vi "Manual Test.vi"() -> ()   [LabVIEW 2019]
uses:
  <vilib>/Gustavo Trejo/PIC Serial Toolkit/Controls/TRISA.ctl
  <vilib>/Gustavo Trejo/PIC Serial Toolkit/Controls/TRISB.ctl
  <vilib>/Gustavo Trejo/PIC Serial Toolkit/Controls/TRISC.ctl
  <vilib>/Gustavo Trejo/PIC Serial Toolkit/Controls/TRISD.ctl
  <vilib>/Gustavo Trejo/PIC Serial Toolkit/Controls/TRISE.ctl
  <vilib>/Gustavo Trejo/PIC Serial Toolkit/Controls/Pin Number.ctl
panel:
  in  "D5":bool
  in  "D4":bool
  out "D3":bool
  out "D2":bool
  in  "Stop Button":bool
  in  "COM":refnum<visa-resource-name>
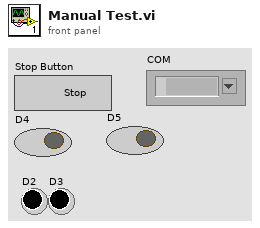
[diagram p1: front panel]
types:
  T1 = typedef "TRISE.ctl" = cluster{"E0":bool, "E1":bool, "E2":bool}
  T2 = typedef "TRISD.ctl" = cluster{"D0":bool, "D1":bool, "D2":bool, "D3":bool, "D4":bool, "D5":bool, "D6":bool, "D7":bool}
  T3 = typedef "TRISC.ctl" = cluster{"C0":bool, "C1":bool, "C2":bool, "C3":bool, "C4":bool, "C5":bool}
  T4 = typedef "TRISB.ctl" = cluster{"B0":bool, "B1":bool, "B2":bool, "B3":bool, "B4":bool, "B5":bool, "B6":bool, "B7":bool}
  T5 = typedef "TRISA.ctl" = cluster{"A0":bool, "A1":bool, "A2":bool, "A3":bool, "A4":bool, "A5":bool, "A6":bool, "A7":bool}
  T6 = typedef "Pin Number.ctl" = enum16{"A0/AN0", "A1/AN1", "A2/AN2", "A3/AN3", "A4", "A5/AN4", "A6", "A7", "B0/AN12", "B1/AN10", "B2/AN8", "B3/AN9", "B4/AN11", "B5/AN13", "B6", "B7", "C0", "C1/PWM2", "C2/PWM1", "C3", "C4", "C5", "D0", "D1", "D2", "D3", "D4", "D5", "D6", "D7", "E0/AN5", "E1/AN6", "E2/AN7"}
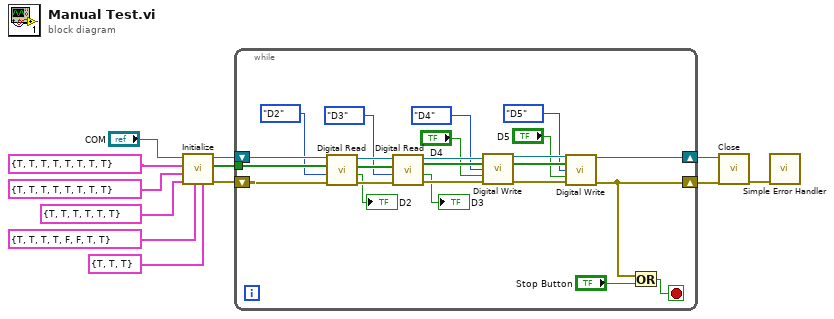
[diagram p0: block diagram]
diagram:
  n1 = call <vilib>:"Initialize.vi"("TRISE E0-E2"=T1 {"E0"=TRUE, "E1"=TRUE, "E2"=TRUE}, "TRISD D0-D7"=T2 {"D0"=TRUE, "D1"=TRUE, "D2"=TRUE, "D3"=TRUE, "D4"=FALSE, "D5"=FALSE, "D6"=TRUE, "D7"=TRUE}, "TRISC C0-C5"=T3 {"C0"=TRUE, "C1"=TRUE, "C2"=TRUE, "C3"=TRUE, "C4"=TRUE, "C5"=TRUE}, "TRISB B0-B7"=T4 {"B0"=TRUE, "B1"=TRUE, "B2"=TRUE, "B3"=TRUE, "B4"=TRUE, "B5"=TRUE, "B6"=TRUE, "B7"=TRUE}, "TRISA A0-A7"=T5 {"A0"=TRUE, "A1"=TRUE, "A2"=TRUE, "A3"=TRUE, "A4"=TRUE, "A5"=TRUE, "A6"=TRUE, "A7"=TRUE}, "VISA Refnum in"="COM") -> ("error out"=w4:errorcluster, "Ports Ref Out"=w5:bool[], "VISA Refnum out"=w6:refnum<visa-resource-name>)  [unwired: 3 in]
  n2 = while {
    tunnel: w5 -> [w35]
    shift-right: [w13] -> w2
    shift-left: w6 -> [w36]
    shift-right: [w14] -> w3
    shift-left: w4 -> [w34]
    stop <- w23 stop-if-true
    n3 = call <vilib>:"Digital Read.vi"("error in (no error)"=w34, "Pin Number"=Pin_Number."D2", "Ports Ref In"=w35, "VISA Refnum in"=w36) -> ("error out"=w33:errorcluster, "Pin State Out"=→"D2":bool, "Ports Ref Out"=w32:bool[], "VISA Refnum out"=w31:refnum<visa-resource-name>)  [unwired: 4 in]
    n4 = call <vilib>:"Digital Read.vi"("error in (no error)"=w33, "Pin Number"=Pin_Number."D3", "Ports Ref In"=w32, "VISA Refnum in"=w31) -> ("error out"=w30:errorcluster, "Pin State Out"=→"D3":bool, "Ports Ref Out"=w28:bool[], "VISA Refnum out"=w29:refnum<visa-resource-name>)  [unwired: 4 in]
    n5 = call <vilib>:"Digital Write.vi"("VISA Refnum in"=w29, "Ports Ref In"=w28, "Pin Number"=Pin_Number."D4", "State Output"="D4", "error in (no error)"=w30) -> ("VISA Refnum out"=w27:refnum<visa-resource-name>, "Ports Ref Out"=w26:bool[], "error out"=w25:errorcluster)  [unwired: 8 in]
    n6 = call <vilib>:"Digital Write.vi"("VISA Refnum in"=w27, "Ports Ref In"=w26, "Pin Number"=Pin_Number."D5", "State Output"="D5", "error in (no error)"=w25) -> ("VISA Refnum out"=w13:refnum<visa-resource-name>, "error out"=w14:errorcluster)  [unwired: 8 in, 1 out]
    n7 = Or(x=w14, y="Stop Button") -> (x .or. y?=w23:bool)
  }
  n8 = call <vilib>:"Close.vi"("error in (no error)"=w3, "VISA Refnum in"=w2) -> ("error out"=w1:errorcluster)  [unwired: 9 in]
  n9 = call <vilib>:"Simple Error Handler.vi"("error in (no error)"=w1) -> ()  [unwired: 4 in, 5 out]
